vi "Close.vi"(8 "error in (no error)":errorcluster, 10 "Force?":bool, 11 "CubeLogger in":refnum<class "CubeLogger.lvclass">) -> (0 "error out":errorcluster, 2 "Repeat?":bool, 3 "CubeLogger out":refnum<class "CubeLogger.lvclass">)   [LabVIEW 2018, in "vis3d.lvlib" / "CubeLogger.lvclass"]
uses:
  CubeLogger.lvclass
  File.ctl
  Dataset.ctl
  Header.ctl
  CubeLogger.lvclass/CubeLogger.ctl
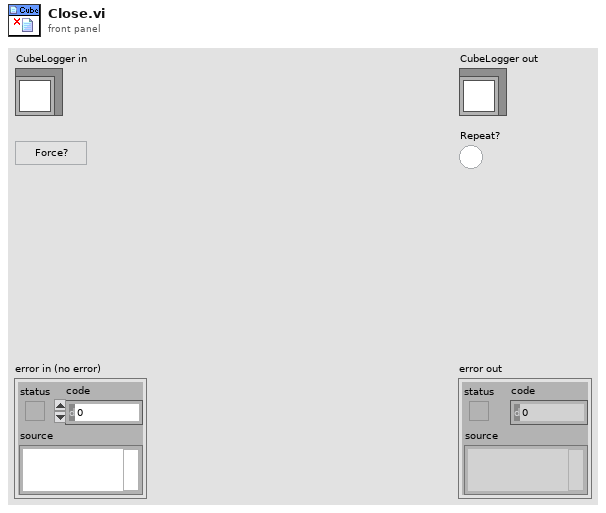
[diagram p1: front panel]
types:
  T1 = cluster{"TotalSteps":i32, "CurrentLog":i32, "Finished?":bool}
  T2 = typedef "vis3d.lvlib/CubeLogger.lvclass/Header.ctl" = cluster{"name":string, "desc":string, "data":variant[], "meta":variant}
  T3 = typedef "vis3d.lvlib/CubeLogger.lvclass/Dataset.ctl" = cluster{"name":string, "path":string, "size":i32[], "type":enum16{"single", "double", "uint8", "uint16", "uint32", "uint64", "int8", "int16", "int32", "int64"}, "mfmt":string, "order":string}
  T4 = typedef "vis3d.lvlib/CubeLogger.lvclass/File.ctl" = cluster{"Name":string, "Folder":path, "Description":string}
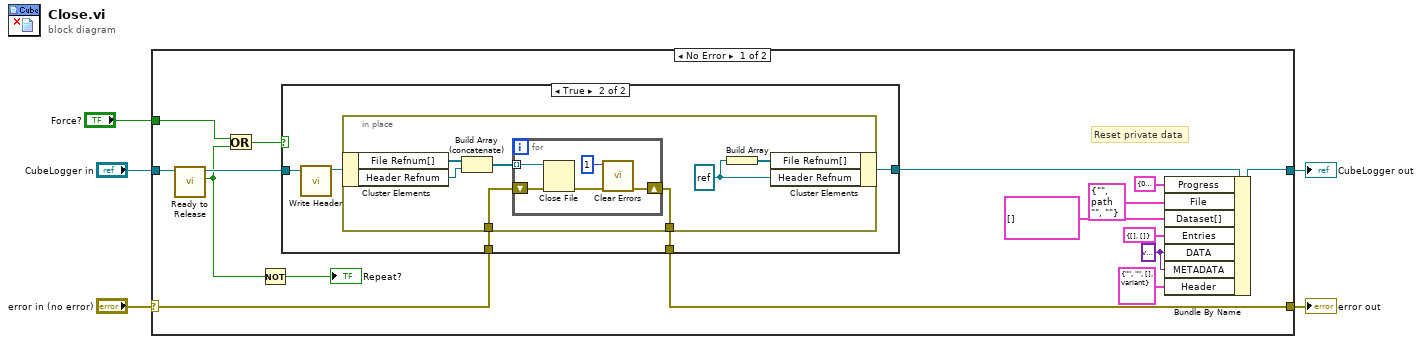
[diagram p0: block diagram]
diagram:
  n1 = case shown="No Error" "error in (no error)" {
    selector: "error in (no error)" -> [w18 w42]
    tunnel: [w17 w42] -> w4
    tunnel: [w12 w41] -> w2
    tunnel: "CubeLogger in" -> [w20 w41]
    tunnel: "Force?" -> [w14 _]
    frame No Error {
      w8 = variant ("DATA")
      # "Reset private data"
      n2 = call "Ready to Release.vi"("CubeLogger in"=w20) -> ("Ready to Release?"=w13:bool, "CubeLogger out"=w19:refnum<class "CubeLogger.lvclass">)  [unwired: 8 in, 1 out]
      n3 = Or(x=w14, y=w13) -> (x .or. y?=w15:bool)
      n4 = Not(x=w13) -> (.not. x?=→"Repeat?":bool)
      n5 = case shown="True" w15 {
        tunnel: [w23 w26] -> w21
        tunnel: w19 -> [w23 w28]
        tunnel: w18 -> [w22 w25]
        tunnel: [w22 w24] -> w17
        frame False {
        }
        frame True {
          n6 = call "Write Header.vi"("CubeLogger in"=w28) -> ("CubeLogger out"=w27:refnum<class "CubeLogger.lvclass">)  [unwired: 8 in, 2 out]
          n7 = in-place {
            in-place-border: w25 -> [w30]
            in-place-border: [w29] -> w24
            w32 = refnum<file> refnum ("Header Refnum")
            n8 = in-place-cluster #1(w27) -> ("File Refnum[]"=w35:refnum<file>[], "Header Refnum"=w34:refnum<file>)
            n9 = Build Array (concatenate)(w35, w34) -> (w31:refnum<file>[])
            n10 = for {
              tunnel: w31 -> [w40] mode=indexing
              shift-right: [w37] -> w29
              shift-left: w30 -> [w38]
              n11 = Close File(refnum=w40, error in=w38) -> (error out=w39:errorcluster)  [unwired: 1 out]
              n12 = call <vilib>:"Clear Errors.vi"("error in (no error)"=w39, "specific error code to clear (0: all)"=1) -> ("error out"=w37:errorcluster)  [unwired: 4 in, 1 out]
            }
            n13 = Build Array(w32) -> (w33:refnum<file>[])
            n14 = in-place-cluster #1("File Refnum[]"=w33, "Header Refnum"=w32) -> (w26:refnum<class "CubeLogger.lvclass">)
          }
        }
      }
      n15 = Bundle By Name(cluster=w21, "Progress"=T1 {"TotalSteps"=0, "CurrentLog"=0, "Finished?"=FALSE}, "File"=T4 {"Name"="", "Folder"=path "", "Description"=""}, "Dataset[]"=T3[] [], "Entries"=cluster{"Name[]":string[], "UUID[]":string[]} {"Name[]"=[], "UUID[]"=[]}, "DATA"=w8, "METADATA"=w8, "Header"=T2 {"name"="", "desc"="", "data"=[], "meta"=variant}) -> (w12:refnum<class "CubeLogger.lvclass">)
    }
    frame Error {
    }
  }
  "error out" <- w4
  "CubeLogger out" <- w2
